vi "Part2-5.vi"() -> ()   [LabVIEW 2015]
uses:
  <vilib>/Analysis/2dsp.llb/1D Convolution (DBL).vi
  <vilib>/Analysis/NI_AALPro.lvlib
panel:
  out "X conv Y":dbl[](graph)
  out "X conv Y":dbl[](array[numeric])
  in  "Y":dbl[](array[numeric])
  in  "X":dbl[](array[numeric])
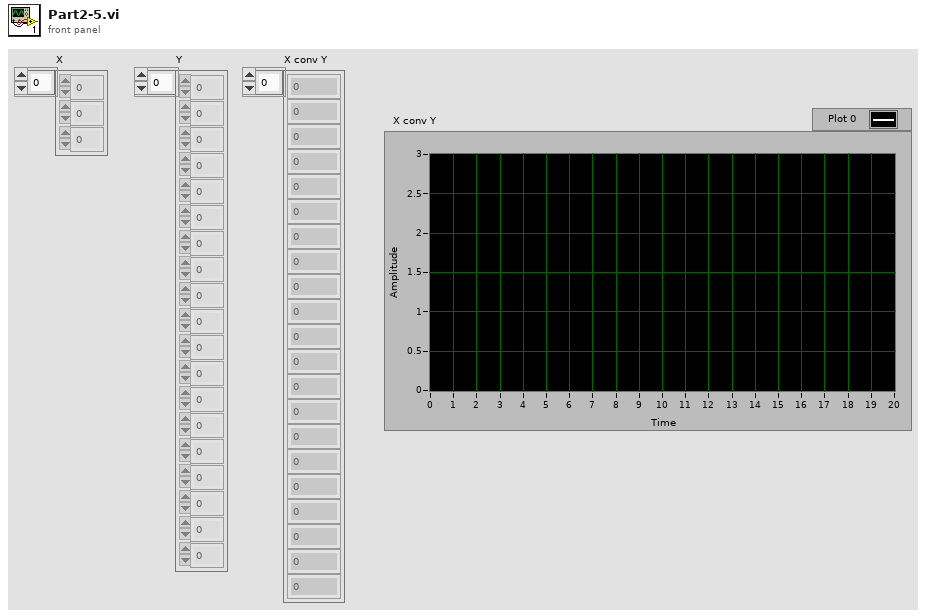
[diagram p1: front panel]
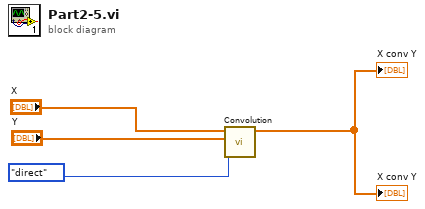
[diagram p0: block diagram]
diagram:
  n1 = call-poly <vilib>:"Convolution.vi"("algorithm"=enum32{"direct", "frequency domain"}."direct", "Y"="Y", "X"="X") -> ("X * Y"=→"X conv Y" →"X conv Y":dbl[])  [unwired: 7 in, 1 out]
